vi "findCOM.vi"(2 "error in (no error)":errorcluster) -> (0 "错误输出":errorcluster, 1 "VISA resource out":refnum<visa-resource-name>)   [LabVIEW 2018]
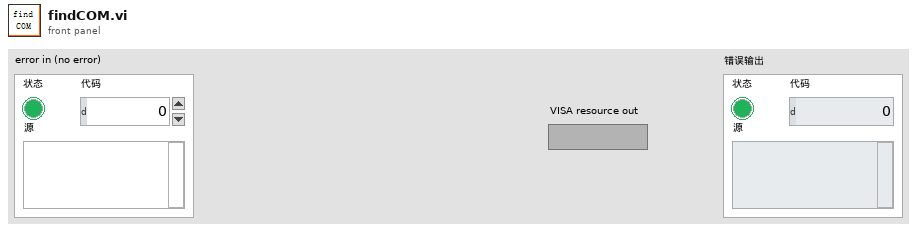
[diagram p1: front panel]
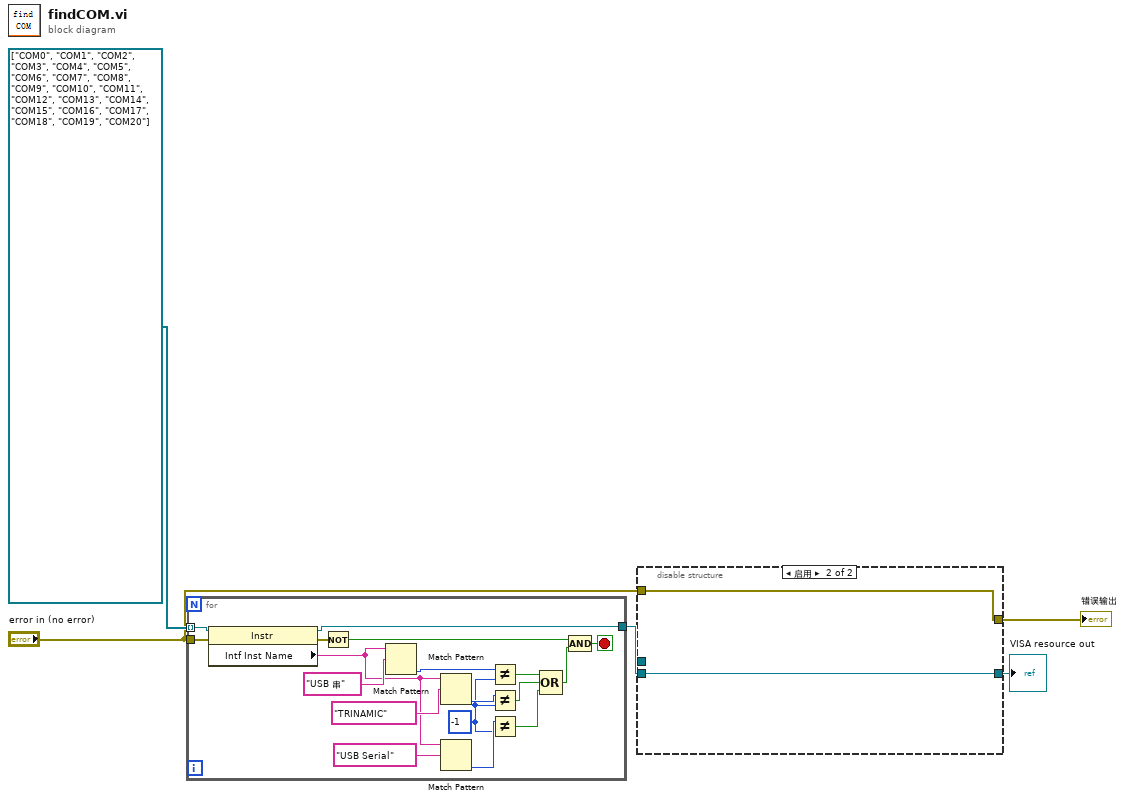
[diagram p0: block diagram]
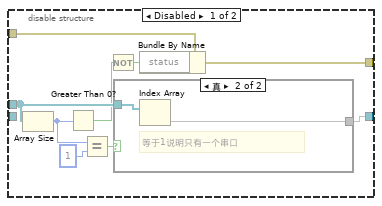
[diagram p2: hidden frame]
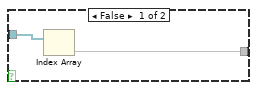
[diagram p3: hidden frame]
diagram:
  n1 = for {
    tunnel: refnum<visa-resource-name>[] ["COM0", "COM1", "COM2", "COM3", "COM4", "COM5", "COM6", "COM7", "COM8", "COM9", "COM10", "COM11", "COM12", "COM13", "COM14", "COM15", "COM16", "COM17", "COM18", "COM19", "COM20"] ("添加的数组") -> [w22] mode=indexing
    tunnel: "error in (no error)" -> [w23]
    tunnel: [w6] -> w1
    stop <- w7 stop-if-true
    w12 = -1 ("y")
    n2 = property class="Instr"(reference=w22, error in=w23) -> (reference out=w6:refnum<visa-resource-name>, error out=w17:errorcluster, "Intf Inst Name"=w15:string)
    n3 = Not(x=w17) -> (.not. x?=w16:bool)
    n4 = Match Pattern(string=w15, regular expression="USB 串" ("正则表达式")) -> (offset past match=w21:i32)  [unwired: 1 in, 3 out]
    n5 = Match Pattern(string=w15, regular expression="TRINAMIC" ("正则表达式")) -> (offset past match=w18:i32)  [unwired: 1 in, 3 out]
    n6 = Match Pattern(string=w15, regular expression="USB Serial" ("正则表达式")) -> (offset past match=w13:i32)  [unwired: 1 in, 3 out]
    n7 = Not Equal?(x=w21, y=w12) -> (x != y?=w11:bool)
    n8 = Not Equal?(x=w18, y=w12) -> (x != y?=w10:bool)
    n9 = Not Equal?(x=w13, y=w12) -> (x != y?=w9:bool)
    n10 = Compound Arithmetic op=OR ("复合运算")(w11, w10, w9) -> (w8:bool)
    n11 = Compound Arithmetic op=AND ("复合运算")(w16, w8) -> (w7:bool)
  }
  n12 = disable-structure shown="启用" {
    disable-tunnel: _ -> [w30 _]
    disable-tunnel: [w29 w37] -> w4
    disable-tunnel: "error in (no error)" -> [w26 w38]
    disable-tunnel: [w24 w38] -> w2
    disable-tunnel: w1 -> [_ w37]
    frame Disabled {
      n13 = Array Size(array=w30) -> (size(s)=w28:i32)
      n14 = Greater Than 0?(x=w28) -> (x > 0?=w27:bool)
      n15 = Equal?(x=w28, y=1) -> (x = y?=w31:bool)
      n16 = Not(x=w27) -> (.not. x?=w25:bool)
      n17 = case shown="真" w31 {
        tunnel: w30 -> [w34 w36]
        tunnel: [w33 w35] -> w29
        frame False {
          n18 = Index Array(array=w34) -> (element=w33)  [unwired: 1 in]
        }
        frame True {
          # "等于1说明只有一个串口"
          n19 = Index Array(array=w36) -> (element=w35)  [unwired: 1 in]
        }
      }
      n20 = Bundle By Name(cluster=w26, "status"=w25) -> (w24:errorcluster)
    }
    frame Enabled {
    }
  }
  "VISA resource out" <- w4
  "错误输出" <- w2
